vi "GetCfgFile.vi"() -> (0 "appended path":path)   [LabVIEW 2025]
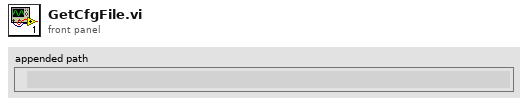
[diagram p1: front panel]
types:
  T1 = enum32{"invalid app kind", "Development System", "Run Time System", "Student Edition", "Embedded LabVIEW", "Evaluation", "Custom"}
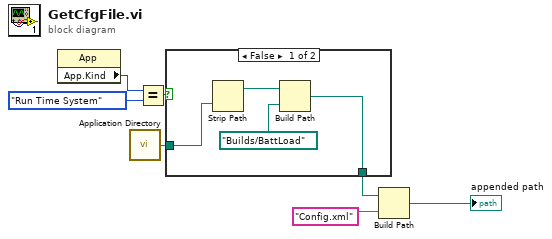
[diagram p0: block diagram]
diagram:
  n1 = property class="App"() -> ("App.Kind"=w6:T1)  [unwired: 2 in, 2 out]
  n2 = call <vilib>:"Application Directory.vi"() -> ("Application Directory"=w3:path)
  n3 = Equal?(x=w6, y=T1."Run Time System") -> (x = y?=w4:bool)
  n4 = case shown="False" w4 {
    tunnel: [w8 w12] -> w2
    tunnel: w3 -> [w11 w12]
    frame False {
      n5 = Strip Path(path=w11) -> (stripped path=w10:path)  [unwired: 1 out]
      n6 = Build Path(base path=w10, name or relative path=path "Builds/BattLoad") -> (appended path=w8:path)
    }
    frame True {
    }
  }
  n7 = Build Path(base path=w2, name or relative path="Config.xml") -> (appended path=→"appended path":path)
